vi "Drive and Climb SS Controls to Commands 2017.vi"(11 "Pilot-CoPilot Controls":T2) -> (3 "Drive/Climb Commands":T1)   [LabVIEW 2016]
uses:
  Robot Control Outputs 2017.ctl
  Drive + Climb Commands 2017.ctl
  Global Variables/Deadband Calibrations.vi
  Global Variables/Robot Status.vi
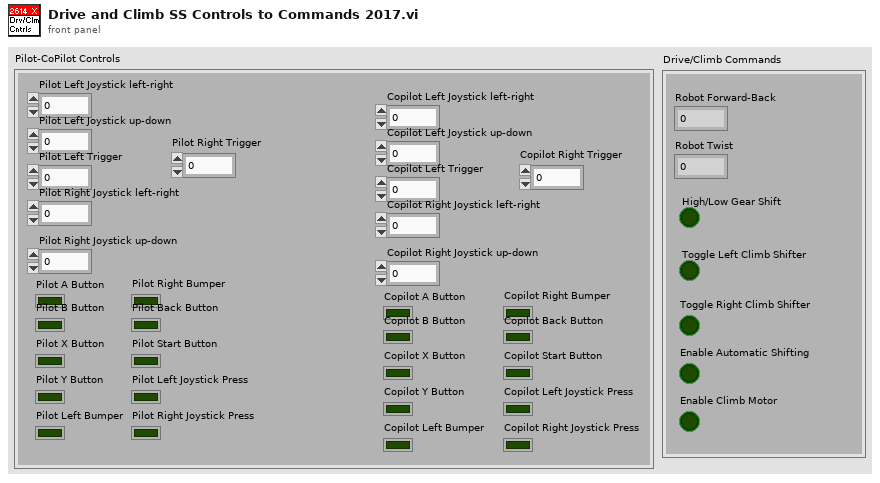
[diagram p1: front panel]
types:
  T1 = typedef "Drive + Climb Commands 2017.ctl" = cluster{"Robot Forward-Back":dbl, "Robot Twist":dbl, "High/Low Gear Shift":bool, "Toggle Left Climb Shifter":bool, "Toggle Right Climb Shifter":bool, "Enable Automatic Shifting":bool, "Enable Climb Motor ":bool}
  T2 = typedef "Robot Control Outputs 2017.ctl" = cluster{"Pilot Left Joystick left-right":dbl, "Pilot Left Joystick up-down":dbl, "Pilot A Button":bool, "Pilot B Button":bool, "Pilot X Button":bool, "Pilot Y Button":bool, "Pilot Left Bumper":bool, "Pilot Right Bumper":bool, "Pilot Back Button":bool, "Pilot Start Button":bool, "Pilot Left Joystick Press":bool, "Pilot Right Joystick Press":bool, "Pilot Left Trigger":dbl, "Pilot Right Joystick left-right":dbl, "Pilot Right Joystick up-down":dbl, "Pilot Right Trigger":dbl, "Copilot Left Joystick left-right":dbl, "Copilot Left Joystick up-down":dbl, "Copilot A Button":bool, "Copilot B Button":bool, "Copilot X Button":bool, "Copilot Y Button":bool, "Copilot Left Bumper":bool, "Copilot Right Bumper":bool, "Copilot Back Button":bool, "Copilot Start Button":bool, "Copilot Left Joystick Press":bool, "Copilot Right Joystick Press":bool, "Copilot Left Trigger":dbl, "Copilot Right Joystick left-right":dbl, "Copilot Right Joystick up-down":dbl, "Copilot Right Trigger":dbl}
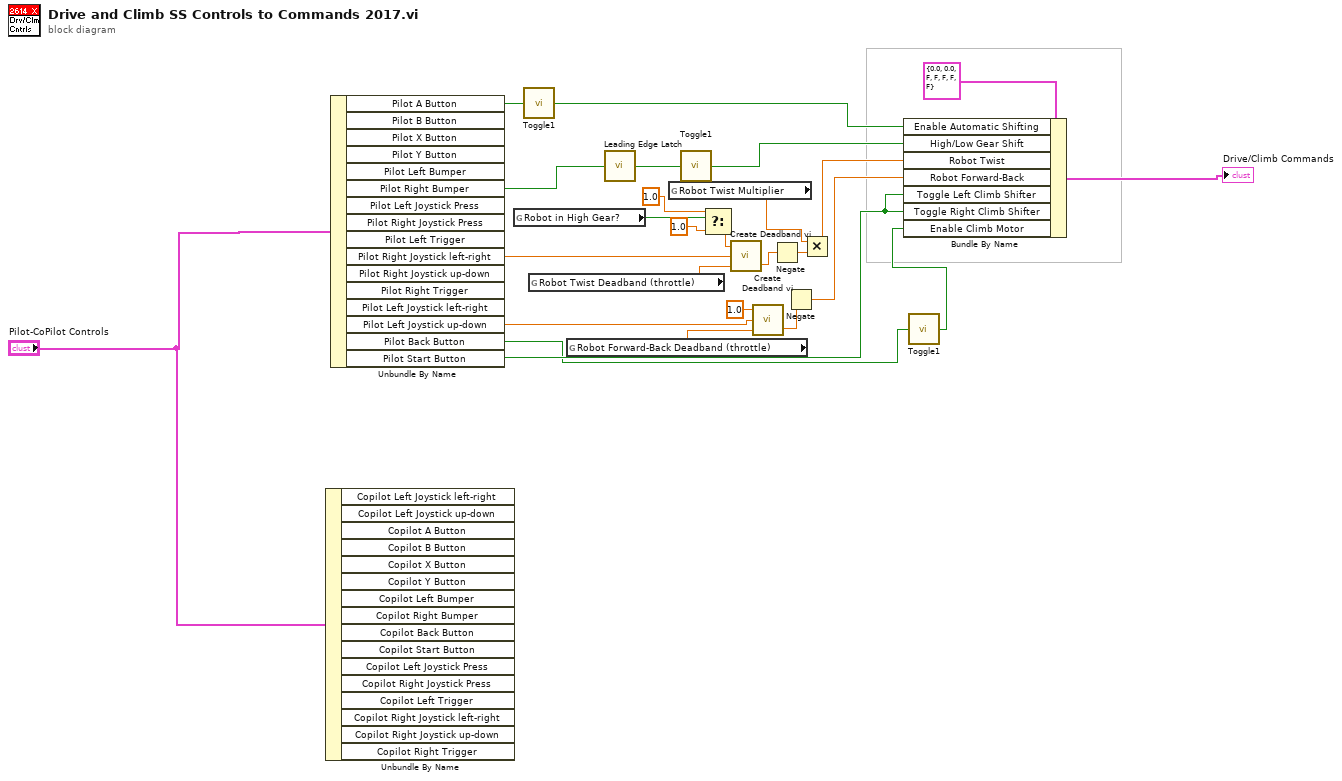
[diagram p0: block diagram]
diagram:
  n1 = Unbundle By Name("Pilot-CoPilot Controls") -> ()  [unwired: 16 out]
  n2 = Unbundle By Name("Pilot-CoPilot Controls") -> ("Pilot A Button"=w15:bool, "Pilot Right Bumper"=w25:bool, "Pilot Right Joystick left-right"=w20:dbl, "Pilot Left Joystick up-down"=w17:dbl, "Pilot Back Button"=w2:bool, "Pilot Start Button"=w3:bool)  [unwired: 10 out]
  n3 = global read "Robot Status.vi" "Robot in High Gear?"() -> (w11:bool)
  n4 = call "Toggle1.vi"("Boolean"=w15) -> ("Driver Switch 2"=w14:bool)
  n5 = global read "Deadband Calibrations.vi" "Robot Twist Deadband (throttle)"() -> (w12:dbl)
  n6 = global read "Deadband Calibrations.vi" "Robot Forward-Back Deadband (throttle)"() -> (w13:dbl)
  n7 = call "Leading Edge Latch.vi"("Input"=w25) -> ("Output"=w7:bool)
  n8 = global read "Deadband Calibrations.vi" "Robot Twist Multiplier"() -> (w4:dbl)
  n9 = call "Toggle1.vi"("Boolean"=w7) -> ("Driver Switch 2"=w24:bool)
  n10 = Select(t=1.0, s=w11, f=1.0) -> (s? t:f=w8:dbl)
  n11 = call "Create Deadband vi.vi"("Input Deadband"=w12, "Input"=w20, "Output Upper Limit"=w8) -> ("Output"=w19:dbl)  [unwired: 1 in]
  n12 = call "Create Deadband vi.vi"("Input Deadband"=w13, "Input"=w17, "Output Upper Limit"=1.0) -> ("Output"=w16:dbl)  [unwired: 1 in]
  n13 = Negate(x=w19) -> (-x=w6:dbl)
  n14 = Negate(x=w16) -> (-x=w23:dbl)
  n15 = Multiply(x=w4, y=w6) -> (x*y=w5:dbl)
  n16 = call "Toggle1.vi"("Boolean"=w2) -> ("Driver Switch 2"=w1:bool)
  n17 = Bundle By Name(cluster=T1 {"Robot Forward-Back"=0.0, "Robot Twist"=0.0, "High/Low Gear Shift"=FALSE, "Toggle Left Climb Shifter"=FALSE, "Toggle Right Climb Shifter"=FALSE, "Enable Automatic Shifting"=FALSE, "Enable Climb Motor "=FALSE} ("Robot Commands"), "Enable Automatic Shifting"=w14, "High/Low Gear Shift"=w24, "Robot Twist"=w5, "Robot Forward-Back"=w23, "Toggle Left Climb Shifter"=w3, "Toggle Right Climb Shifter"=w3, "Enable Climb Motor"=w1) -> (→"Drive/Climb Commands":T1)
